vi "HW_GEN - Update Para In Tree to ChanCFG Variable.vi"(7 "Para In Tree":cluster{"ColHdrs":string[], "Items":string[][]}, 9 "Paravalues[]":string[][](array[string]), 10 "ParaNames[]":string[](array[string])) -> (1 "Paravalues[]":string[][](array[string]))   [LabVIEW 2016]
doc: "对tree中与ChanCFG中同名参数进行值更新；\nChanCFG中的参数有可能比在tree控件上显示的参数要多。"
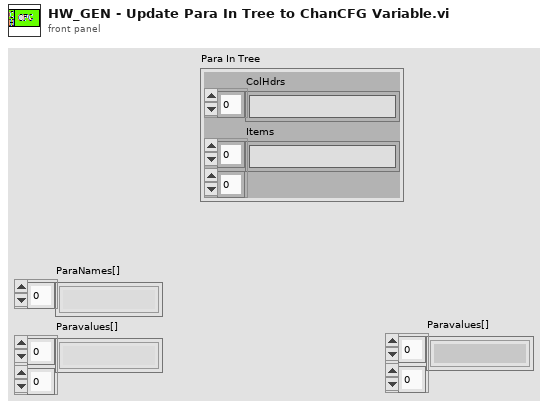
[diagram p1: front panel]
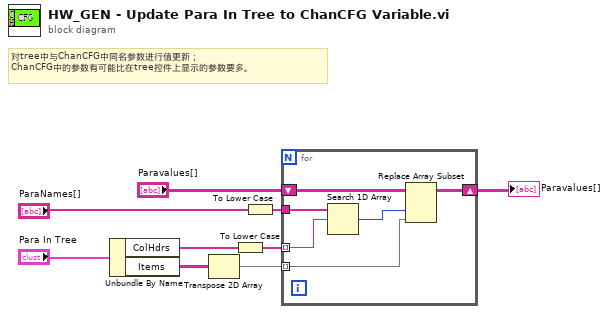
[diagram p0: block diagram]
diagram:
  # "对tree中与ChanCFG中同名参数进行值更新；\nChanCFG中的参数有可能比在tree控件上显示的参数要多。"
  n1 = Unbundle By Name("Para In Tree") -> ("ColHdrs"=w8:string[], "Items"=w5:string[][])
  n2 = Transpose 2D Array(2D array=w5) -> (transposed array=w4:string[][])
  n3 = To Lower Case(string=w8) -> (all lower case string=w7:string[])
  n4 = To Lower Case(string="ParaNames[]") -> (all lower case string=w6:string[])
  n5 = for {
    tunnel: w7 -> [w14] mode=indexing
    tunnel: w6 -> [w15]
    tunnel: w4 -> [w11] mode=indexing
    shift-right: [w10] -> w1
    shift-left: "Paravalues[]" -> [w13]
    n6 = Search 1D Array(1D array=w15, element=w14) -> (index of element=w12:i32)  [unwired: 1 in]
    n7 = Replace Array Subset(array=w13, new element=w11, index (col)=w12) -> (w10:string[][])  [unwired: 1 in]
  }
  "Paravalues[]" <- w1
